vi "SwerveDriveV2.vi"() -> ()   [LabVIEW 2016]
panel:
  in  "Z":dbl
  in  "Y":dbl
  in  "X":dbl
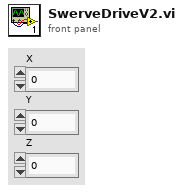
[diagram p1: front panel]
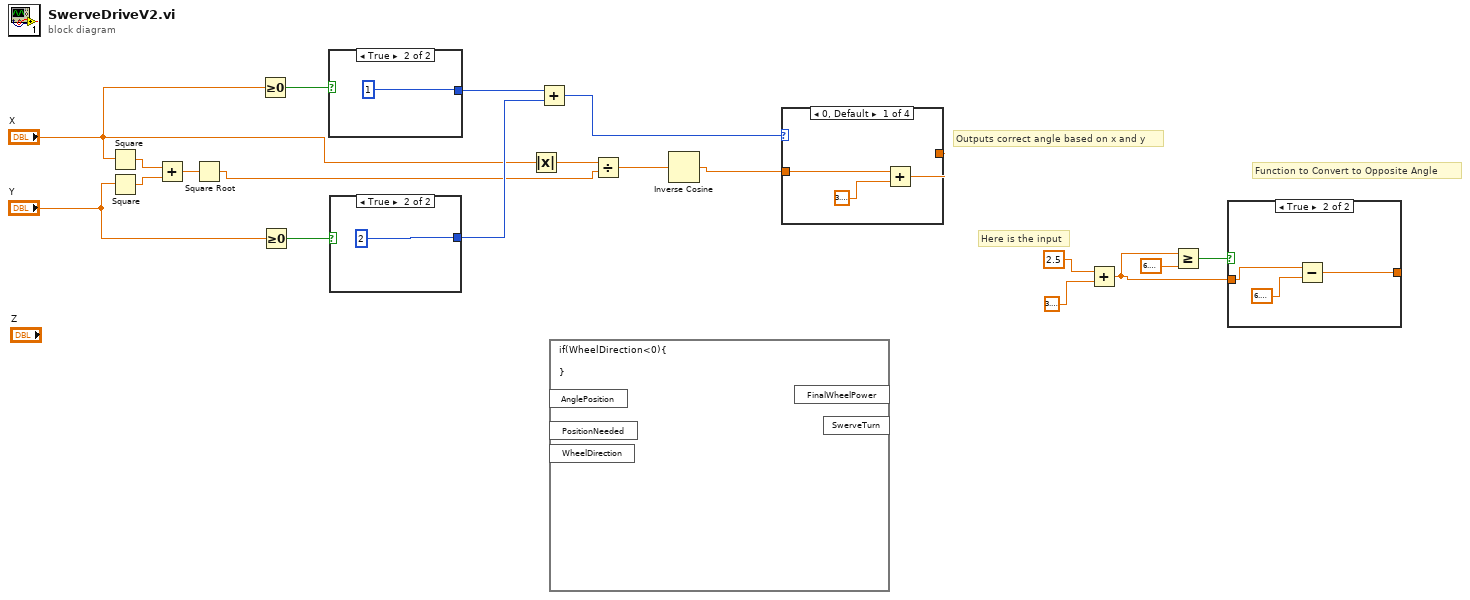
[diagram p0: block diagram]
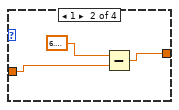
[diagram p3: hidden frame]
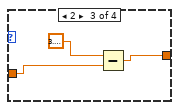
[diagram p4: hidden frame]
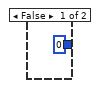
[diagram p6: hidden frame]
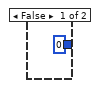
[diagram p7: hidden frame]
diagram:
  # "Function to Convert to Opposite Angle"
  # "Outputs correct angle based on x and y"
  # "Here is the input"
  n1 = Square(x="X") -> (x^2=w19:dbl)
  n2 = Square(x="Y") -> (x^2=w18:dbl)
  n3 = Add(x=w19, y=w18) -> (x+y=w17:dbl)
  n4 = Square Root(x=w17) -> (sqrt(x)=w8:dbl)
  n5 = Greater Or Equal To 0?(x="X") -> (x >= 0?=w15:bool)
  n6 = Greater Or Equal To 0?(x="Y") -> (x >= 0?=w14:bool)
  n7 = case shown="True" w15 {
    tunnel: [0 1] -> w13
    frame False {
    }
    frame True {
    }
  }
  n8 = case shown="True" w14 {
    tunnel: [0 2] -> w12
    frame False {
    }
    frame True {
    }
  }
  n9 = Absolute Value(x="X") -> (abs(x)=w9:dbl)
  n10 = Add(x=w13, y=w12) -> (x+y=w11:i32)
  n11 = formula code="if(WheelDirection<0){\n\n}"() -> ()  [unwired: 3 in, 2 out]
  n12 = Divide(x=w9, y=w8) -> (x/y=w7:dbl)
  n13 = Inverse Cosine(1:w7) -> (0:w6:dbl)
  n14 = case shown="0, Default" w11 {
    tunnel: w6 -> [w25 w28 w31 w33]
    tunnel: [w24 w27 w30 w33] -> _
    frame 0, Default {
      n15 = Add(x=w25, y=3.141592653589793) -> (x+y=w24:dbl)
    }
    frame 1 {
      n16 = Subtract(x=6.283185307179586, y=w28) -> (x-y=w27:dbl)
    }
    frame 2 {
      n17 = Subtract(x=3.141592653589793, y=w31) -> (x-y=w30:dbl)
    }
    frame 3 {
    }
  }
  n18 = Add(x=2.5, y=3.141592653589793) -> (x+y=w1:dbl)
  n19 = Greater Or Equal?(x=w1, y=6.283185307179586) -> (x >= y?=w2:bool)
  n20 = case shown="True" w2 {
    tunnel: w1 -> [w34 w37]
    tunnel: [w34 w35] -> _
    frame False {
    }
    frame True {
      n21 = Subtract(x=w37, y=6.283185307179586) -> (x-y=w35:dbl)
    }
  }
